vi "Get Attribute as JSON.vi"(8 "error in":errorcluster, 10 "Attribute":string, 11 "Config from EXCEL in":refnum<class "Config from EXCEL.lvclass">) -> (0 "error out":errorcluster, 2 "<JSON>":string, 3 "Config from EXCEL out":refnum<class "Config from EXCEL.lvclass">)   [LabVIEW 2025, in "Config from EXCEL.lvclass"]
uses:
  Config from EXCEL.lvclass
  Config from EXCEL.lvclass/Config from EXCEL.ctl
  <vilib>/JDP Science/JSONtext/JSONtext.lvlib
  Open-Xml-LabVIEW/Source/Open Xml.lvlib
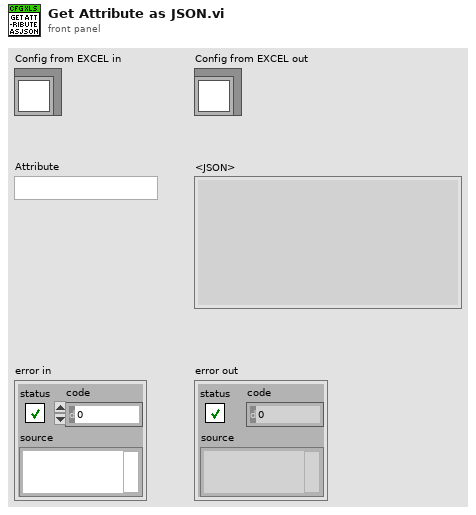
[diagram p1: front panel]
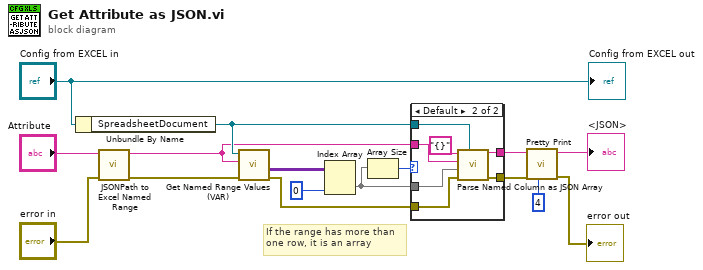
[diagram p0: block diagram]
diagram:
  # "If the range has more than\none row, it is an array"
  n1 = Unbundle By Name("Config from EXCEL in") -> ("SpreadsheetDocument"=w6:refnum<k24>)
  n2 = call "JSONPath to Excel Named Range.vi"("error in"="error in", "JSONPath"="Attribute") -> ("error out"=w13:errorcluster, "Named Range"=w3:string)  [unwired: 8 in]
  n3 = call "Get Named Range Values (VAR).vi"("error in"=w13, "Named Range Identifier"=w3, "SpreadsheetDoc in"=w6) -> ("error out"=w10:errorcluster, "Cells"=w12:variant[][])  [unwired: 6 in, 1 out]
  n4 = Index Array(array=w12, index (col)=0) -> (element=w2:variant[])  [unwired: 1 in]
  n5 = Array Size(array=w2) -> (size(s)=w1:i32)
  n6 = case shown="Default" w1 {
    tunnel: w10 -> [w17 w24]
    tunnel: w6 -> [_ w23]
    tunnel: [w17 w21] -> w5
    tunnel: [_ w20] -> w4
    tunnel: w3 -> [_ w19]
    tunnel: w2 -> [_ w18]
    frame 1 {
    }
    frame Default {
      n7 = call "Parse Named Column as JSON Array.vi"("SpreadsheetDocument in"=w23, "error in"=w24, "Cells"=w18, "Named Range"=w19, "<JSON>"="{}") -> ("error out"=w21:errorcluster, "<JSON> out"=w20:string)  [unwired: 5 in]
    }
  }
  n8 = call <vilib>:"Pretty Print.vi"("Pretty Print Levels"=4, "error in (no error)"=w5, "JSON"=w4) -> ("error out"=→"error out":errorcluster, "<JSON>"=→"<JSON>":string)  [unwired: 6 in, 1 out]
  "Config from EXCEL out" <- "Config from EXCEL in"
